vi "close config file.vi"(8 "error in (no error)":errorcluster, 10 "write file if changed (T)":bool=TRUE, 11 "Refnum in":T1) -> (0 "error out":errorcluster)   [LabVIEW 2024, in "API Config Files Management.lvlib"]
doc: "This function closes the currently opened configuration .ini file, destroying the associated Refnum. It ensures that the file is properly closed, and no further operations can be performed until the file is reopened."
uses:
  API Config Files Management.lvlib
  <vilib>/Utility/config.llb/NI_LVConfig.lvlib
  <vilib>/Utility/config.llb/Config Data RefNum.ctl
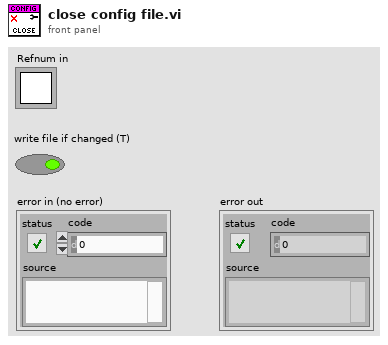
[diagram p1: front panel]
types:
  T1 = typedef "NI_LVConfig.lvlib/Config Data RefNum.ctl" = refnum<k1>
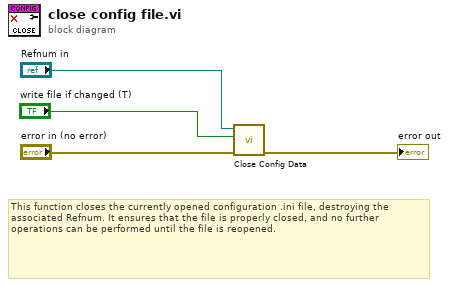
[diagram p0: block diagram]
diagram:
  # "This function closes the currently opened configuration .ini file, destroying the associated Refnum. It ensures that the file is properly closed, and no further operations can be performed until the file is reopened."
  n1 = call <vilib>:"Close Config Data.vi"("error in (no error)"="error in (no error)", "write file if changed (T)"="write file if changed (T)", "refnum"="Refnum in") -> ("error out"=→"error out":errorcluster)  [unwired: 7 in, 1 out]
